vi "linear interpolation iiii- complex -- build matrix.vi"(11 "N":i32) -> (2 "Inverse Matrix":T1)   [LabVIEW 2020]
uses:
  <vilib>/Analysis/Matrix/Datatypes/RealMatrix.ctl
  <vilib>/Analysis/Matrix/Numeric/Conversions/Array To Matrix - RA2.vi
  <vilib>/Analysis/baseanly.llb/Real Inverse Matrix.vi
  <vilib>/Analysis/Matrix/NI_Matrix.lvlib
  <vilib>/Analysis/NI_AALBase.lvlib
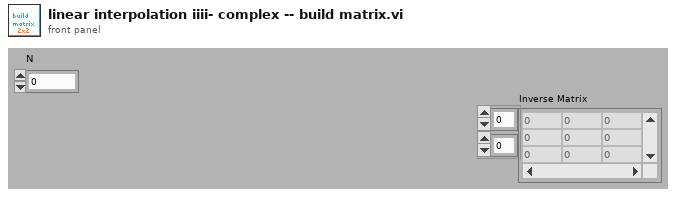
[diagram p1: front panel]
types:
  T1 = typedef "NI_Matrix.lvlib/RealMatrix.ctl" = dbl[][]
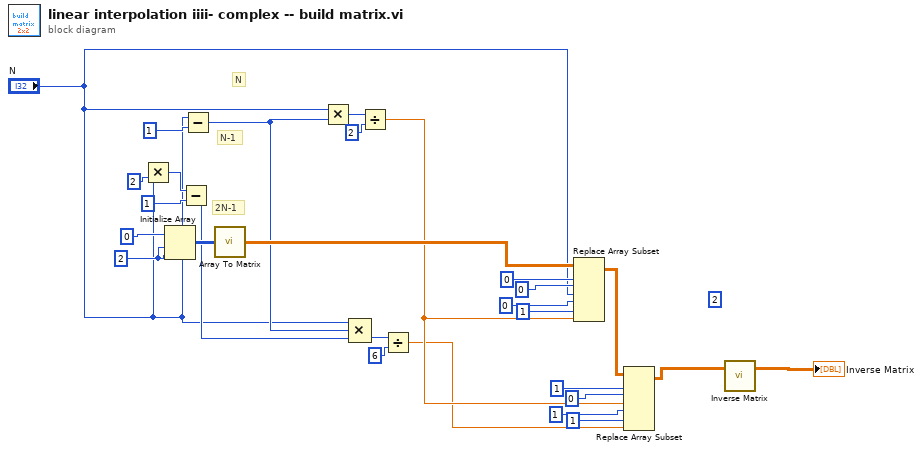
[diagram p0: block diagram]
diagram:
  (unwired) 2 ("n")
  w23 = 2 ("n")
  # "2N-1"
  # "N-1"
  # "N"
  n1 = Multiply(x="N", y=2 ("n")) -> (x*y=w25:i32)
  n2 = Initialize Array(0 ("n"), w23, w23) -> (w22:i32[][])
  n3 = Subtract(x=w25, y=1 ("n")) -> (x-y=w14:i32)
  n4 = Subtract(x="N", y=1 ("n")) -> (x-y=w13:i32)
  n5 = call-poly <vilib>:"Array To Matrix.vi"("Real 2D Array"=w22) -> ("Real Matrix"=w21:T1)
  n6 = Multiply(x="N", y=w13) -> (x*y=w18:i32)
  n7 = Compound Arithmetic op=MULTIPLY("N", w13, w14) -> (w15:i32)
  n8 = Divide(x=w18, y=2 ("n")) -> (x/y=w5:dbl)
  n9 = Divide(x=w15, y=6 ("n")) -> (x/y=w4:dbl)
  n10 = Replace Array Subset(array=w21, new element #1="N", index (row) #1=0 ("n"), index (col) #1=0 ("n"), new element #2=w5, index (row) #2=0 ("n"), index (col) #2=1 ("n")) -> (w6:T1)
  n11 = Replace Array Subset(array=w6, new element #1=w5, index (row) #1=1 ("n"), index (col) #1=0 ("n"), new element #2=w4, index (row) #2=1 ("n"), index (col) #2=1 ("n")) -> (w1:T1)
  n12 = call-poly <vilib>:"Inverse Matrix.vi"("Input Matrix"=w1) -> ("Inverse Matrix"=→"Inverse Matrix":T1)  [unwired: 1 in, 1 out]
